vi "Energize.vi"(8 "error in (no error)":errorcluster, 11 "CIFCorePlugin in":refnum<class "CIFCorePlugin.lvclass">) -> (0 "error out":errorcluster, 3 "CIFCorePlugin out":refnum<class "CIFCorePlugin.lvclass">)   [LabVIEW 2021, in "CIFCorePlugin.lvclass"]
uses:
  CIFCorePlugin.lvclass
  <vilib>/Platform/TimedLoop/XDataNode/timing_clust.ctl
  <vilib>/Platform/TimedLoop/XDataNode/nitl_modes.ctl
  <vilib>/Platform/TimedLoop/XDataNode/wakeup.ctl
  <vilib>/Platform/TimedLoop/XDataNode/XDataNode.xnode
  CIFCorePlugin.lvclass/CIFCorePlugin.ctl
  <vilib>/Platform/TimedLoop/XDataNode/XDNodeRunTimeDep.lvlib
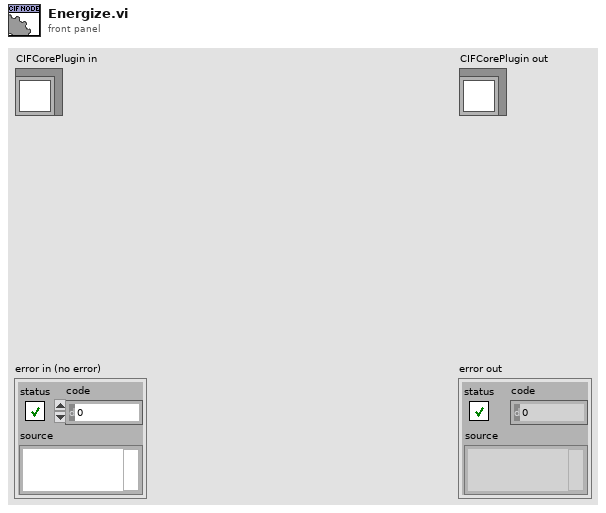
[diagram p1: front panel]
types:
  T1 = typedef "XDNodeRunTimeDep.lvlib/timing_clust.ctl" = cluster{"Expected End [f-1]":u64, "Actual End [f-1]":u64, "Finished Late? [f-1]":bool, "Expected End [i-1]":u64, "Actual End [i-1]":u64, "Finished Late? [i-1]":bool, "Expected Start [i]":u64, "Actual Start [i]":u64, "Expected Start [f]":u64, "Actual Start [f]":u64, "Source Name":string, "Structure Name":string, "Period":i64, "Deadline":i64, "Offset":i64, "Start":i64, "Priority":i32, "Timeout":i32, "Mode":T2, "Wakeup Reason":T3, "Error":errorcluster, "Source Type":string, "Secondary Source Type":string, "Global End Time":u64, "Global Start Time":u64, "Frame Duration":u64, "Iteration Duration":u64, "Assigned CPU":i32, "I/O Scan Engine Mode":u32}
  T2 = typedef "XDNodeRunTimeDep.lvlib/nitl_modes.ctl" = enum32{"No Change", "Process missed periods, maintain original phase", "Discard missed periods, maintain original phase", "Process missed periods, ignore original phase", "Discard missed periods, ignore original phase"}
  T3 = typedef "XDNodeRunTimeDep.lvlib/wakeup.ctl" = enum32{"Normal", "Aborted", "Asynchronous wakeup", "Timing source error", "Timed loop error", "Timeout"}
  T4 = typedef "CIFCorePlugin.lvclass/Prepare State Logic.ctl" = enum16{"Listen", "Prepare", "Error", "Destroy"}
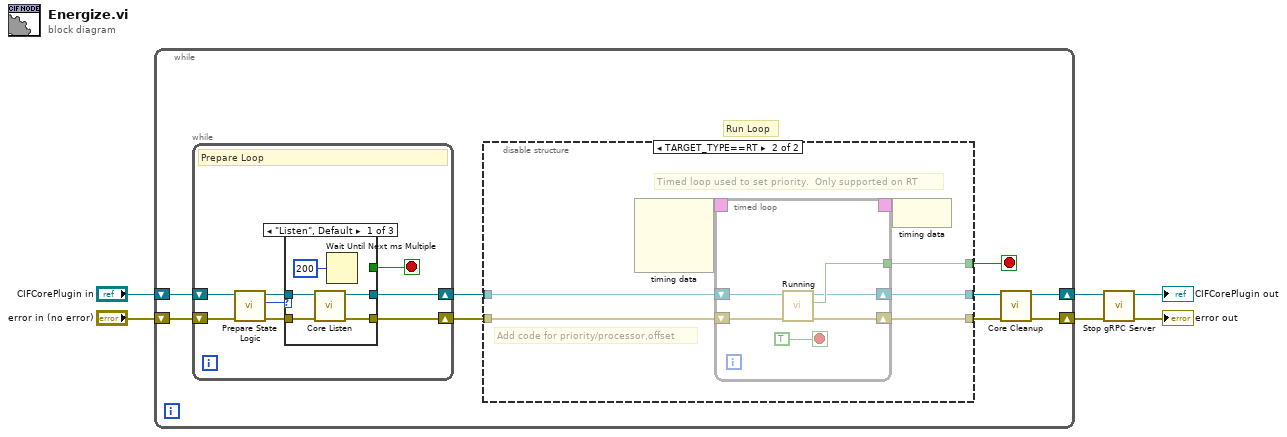
[diagram p0: block diagram]
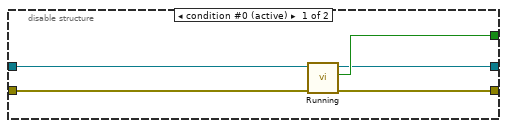
[diagram p2: hidden frame]
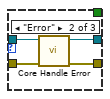
[diagram p3: hidden frame]
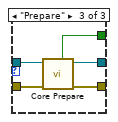
[diagram p4: hidden frame]
diagram:
  n1 = while {
    shift-right: [w8] -> w4
    shift-left: "CIFCorePlugin in" -> [w15]
    shift-right: [w7] -> w3
    shift-left: "error in (no error)" -> [w14]
    stop <- w11 stop-if-true
    # "Run Loop"
    n2 = while {
      shift-right: [w45] -> w13
      shift-left: w15 -> [w44]
      shift-right: [w39] -> w12
      shift-left: w14 -> [w40]
      stop <- w38 stop-if-true
      # "Prepare Loop"
      n3 = call "Prepare State Logic.vi"("error in (no error)"=w40, "CIFCorePlugin in"=w44) -> ("error out"=w41:errorcluster, "Prepare State Logic"=w42:T4, "CIFCorePlugin out"=w43:refnum<class "CIFCorePlugin.lvclass">)  [unwired: 7 in]
      n4 = case shown="\"Listen\", Default" w42 {
        tunnel: [w47 w54 w59] -> w45
        tunnel: w43 -> [w50 w51 w55]
        tunnel: w41 -> [w49 w52 w56]
        tunnel: [w48 w53 w58] -> w39
        tunnel: [_ _ w57] -> w38
        frame "Listen", Default {
          n5 = call "Core Listen.vi"("error in (no error)"=w49, "CIFTemplateNode in"=w50) -> ("error out"=w48:errorcluster, "CIFTemplateNode out"=w47:refnum<class "CIFCorePlugin.lvclass">)  [unwired: 8 in]
          n6 = Wait Until Next ms Multiple(millisecond multiple=u32 200) -> ()  [unwired: 1 out]
        }
        frame "Error" {
          n7 = call "Core Handle Error.vi"("error in (no error)"=w52, "CIFTemplateNode in"=w51) -> ("error out"=w53:errorcluster, "CIFTemplateNode out"=w54:refnum<class "CIFCorePlugin.lvclass">)  [unwired: 8 in]
        }
        frame "Prepare" {
          n8 = call "Core Prepare.vi"("error in (no error)"=w56, "CIFTemplateNode in"=w55) -> ("error out"=w58:errorcluster, "CIFTemplateNode out"=w59:refnum<class "CIFCorePlugin.lvclass">, "Transition to Run"=w57:bool)  [unwired: 7 in]
        }
      }
    }
    n9 = disable-structure shown="TARGET_TYPE==RT" {
      disable-tunnel: w13 -> [w20 w25]
      disable-tunnel: w12 -> [w19 w24]
      disable-tunnel: [w18 w23] -> w11
      disable-tunnel: [w17 w22] -> w10
      disable-tunnel: [w16 w21] -> w9
      frame condition #0 (active) {
        n10 = call "Running.vi"("error in (no error)"=w19, "CIFCorePlugin in"=w20) -> ("error out"=w16:errorcluster, "Destroy"=w18:bool, "CIFCorePlugin out"=w17:refnum<class "CIFCorePlugin.lvclass">)  [unwired: 7 in]
      }
      frame condition #1 {
        # "Add code for priority/processor,offset"
        # "Timed loop used to set priority.  Only supported on RT"
        n11 = node-c288() -> (w27:T1)  [unwired: 3 in]
        n12 = timed-loop {
          timing: w27 -> [_]
          timing-out: [_] -> w26
          shift-right: [w29] -> w22
          shift-left: w25 -> [w32]
          shift-right: [w28] -> w21
          shift-left: w24 -> [w31]
          tunnel: [w30] -> w23
          stop <- TRUE stop-if-true
          n13 = call "Running.vi"("error in (no error)"=w31, "CIFCorePlugin in"=w32) -> ("error out"=w28:errorcluster, "Destroy"=w30:bool, "CIFCorePlugin out"=w29:refnum<class "CIFCorePlugin.lvclass">)  [unwired: 7 in]
        }
        n14 = node-c288(w26) -> ()
      }
    }
    n15 = call "Core Cleanup.vi"("error in (no error)"=w9, "CIFTemplateNode in"=w10) -> ("error out"=w7:errorcluster, "CIFTemplateNode out"=w8:refnum<class "CIFCorePlugin.lvclass">)  [unwired: 8 in]
  }
  n16 = call "Stop gRPC Server.vi"("error in (no error)"=w3, "CIFCorePlugin in"=w4) -> ("error out"=→"error out":errorcluster, "CIFCorePlugin out"=→"CIFCorePlugin out":refnum<class "CIFCorePlugin.lvclass">)  [unwired: 8 in]
